vi "TSPopup.Set Font Size.vi"(8 "error in (no error)":errorcluster, 9 "Font Size":u32, 11 "Popup Cluster Ref":refnum<vi>) -> (0 "error out":errorcluster, 3 "dup ref out":refnum<vi>)   [LabVIEW 2016, in "TSPopup.lvlib" / "TSPopup.lvclass"]
doc: "Sets the font size of the text popup controls.\n\nType Sensitive Popup \nCopyright © 2007, J. David Saunders\nAll rights reserved."
uses:
  <userlib>/TSPopup/TSPopup.lvclass
  <userlib>/TSPopup/TSPopup.Data Type.ctl
panel:
  # "Type Sensitive Popup \nCopyright © 2007, J. David Saunders\nAll rights reserved."
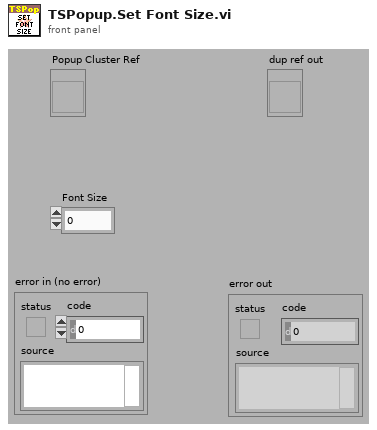
[diagram p1: front panel]
types:
  T1 = typedef "TSPopup.lvlib/TSPopup.lvclass/TSPopup.Data Type.ctl" = enum16{"Unkown", "NO POPUP", "String", "Integer", "Float", "Color", "Boolean", "Ring", "Captioned String", "Captioned Integer", "Button Color", "2 Int Cluster", "4 Int Cluster", "check"}
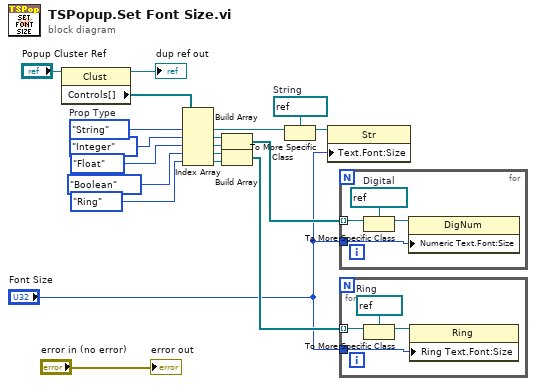
[diagram p0: block diagram]
diagram:
  w17 = refnum<vi> refnum  # String
  w19 = TSPopup.Data_Type."String"  # Prop Type
  n1 = property class="Clust"(reference="Popup Cluster Ref") -> (reference out=→"dup ref out":refnum<vi>, "Controls[]"=w3:refnum<vi>[])  [unwired: 1 in, 1 out]
  n2 = Index Array(array=w3, index #1=w19, index #2=TSPopup.Data_Type."Integer" ("Prop Type"), index #3=TSPopup.Data_Type."Float" ("Prop Type"), index #4=TSPopup.Data_Type."Boolean" ("Prop Type"), index #5=TSPopup.Data_Type."Ring" ("Prop Type")) -> (element #1=w18:refnum<vi>, element #2=w13:refnum<vi>, element #3=w12:refnum<vi>, element #4=w8:refnum<vi>, element #5=w7:refnum<vi>)
  n3 = Build Array(w13, w12) -> (w11:refnum<vi>[])
  n4 = Build Array(w8, w7) -> (w6:refnum<vi>[])
  n5 = To More Specific Class(target class=w17, reference=w18) -> (specific class reference=w16:refnum<vi>)  [unwired: 1 in, 1 out]
  n6 = property class="Str"(reference=w16, "Text.Font:Size"="Font Size") -> ()  [unwired: 1 in, 2 out]
  n7 = for {
    tunnel: w11 -> [w21] mode=indexing
    tunnel: "Font Size" -> [w20]
    w22 = refnum<vi> refnum  # Digital
    n8 = To More Specific Class(target class=w22, reference=w21) -> (specific class reference=w23:refnum<vi>)  [unwired: 1 in, 1 out]
    n9 = property class="DigNum"(reference=w23, "Numeric Text.Font:Size"=w20) -> ()  [unwired: 1 in, 2 out]
  }
  n10 = for {
    tunnel: w6 -> [w25] mode=indexing
    tunnel: "Font Size" -> [w24]
    w26 = refnum<vi> refnum  # Ring
    n11 = To More Specific Class(target class=w26, reference=w25) -> (specific class reference=w27:refnum<vi>)  [unwired: 1 in, 1 out]
    n12 = property class="Ring"(reference=w27, "Ring Text.Font:Size"=w24) -> ()  [unwired: 1 in, 2 out]
  }
  "error out" <- "error in (no error)"
